vi "Version To Dotted String.vi"(1 "Version":T1) -> (0 "String Version":string)   [LabVIEW 2017]
uses:
  <vilib>/_xctls/Version.ctl
  <vilib>/_xctls/XControlSupport.lvlib
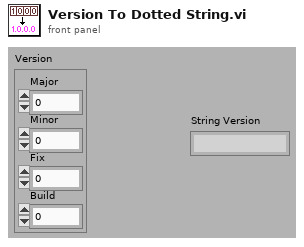
[diagram p1: front panel]
types:
  T1 = typedef "XControlSupport.lvlib/Version.ctl" = cluster{"Major":u16, "Minor":u16, "Fix":u16, "Build":u16}
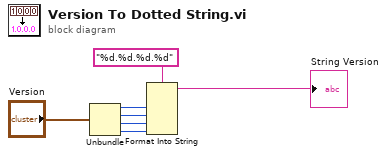
[diagram p0: block diagram]
diagram:
  n1 = Unbundle("Version") -> ("Major"=w3:u16, "Minor"=w4:u16, "Fix"=w5:u16, "Build"=w6:u16)
  n2 = Format Into String(format string="%d.%d.%d.%d", w3, w4, w5, w6) -> (resulting string=→"String Version":string)  [unwired: 2 in, 1 out]
